vi "load_stepfile.vi"(8 "error in (no error)":errorcluster, 11 "_delayStageBase in":refnum<class "_delayStageBase.lvclass">) -> (0 "error out":errorcluster, 3 "_delayStageBase out":refnum<class "_delayStageBase.lvclass">)   [LabVIEW 2018, in "_delayStageBase.lvclass"]
uses:
  _delayStageBase.lvclass
  <vilib>/Utility/file.llb/Read Delimited Spreadsheet (DBL).vi
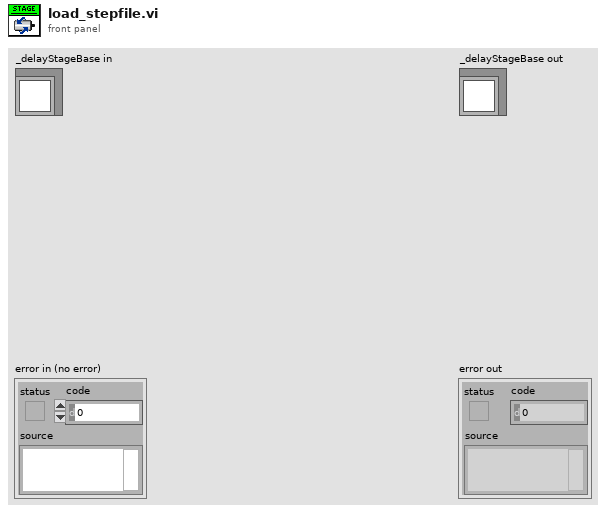
[diagram p1: front panel]
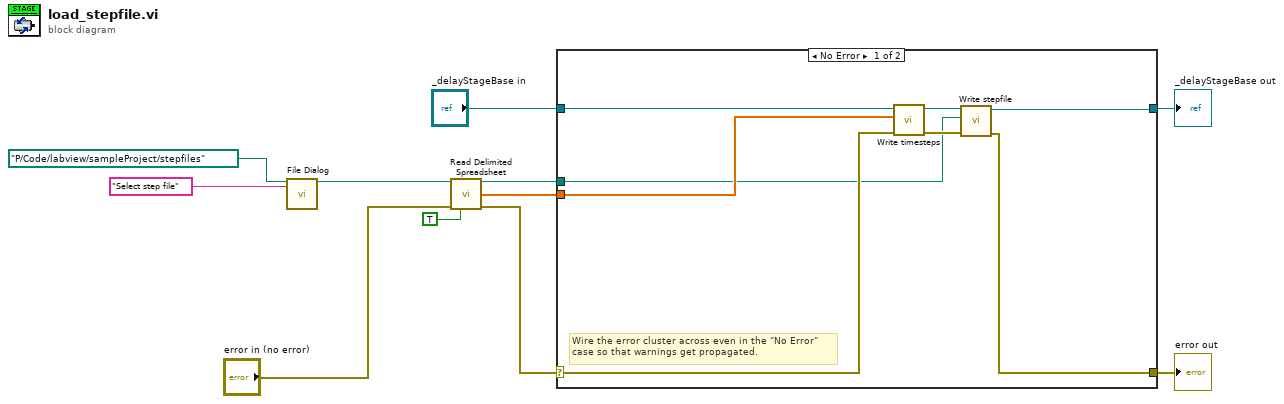
[diagram p0: block diagram]
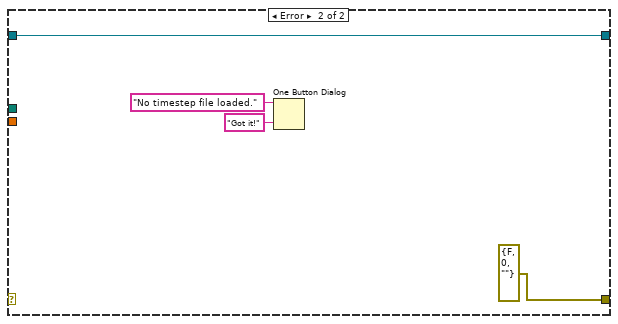
[diagram p2: hidden frame]
diagram:
  n1 = call "File Dialog"("start path"=path "P:/Code/labview/sampleProject/stepfiles", "prompt"="Select step file") -> ("selected path"=w3:path)  [unwired: 10 in, 3 out]
  n2 = call-poly <vilib>:"Read Delimited Spreadsheet.vi"("file path (dialog if empty)"=w3, "error in (no error)"="error in (no error)", "transpose? (F)"=TRUE) -> ("new file path (Not A Path if cancelled)"=w4:path, "first row"=w8:dbl[], "error out"=w5:errorcluster)  [unwired: 7 in, 3 out]
  n3 = case shown="No Error" w5 {
    selector: w5 -> [w18 _]
    tunnel: [w13 errorcluster {"status"=FALSE, "code"=0, "source"=""} ("error out")] -> w11
    tunnel: [w15 w23] -> w9
    tunnel: "_delayStageBase in" -> [w19 w23]
    tunnel: w8 -> [w17 _]
    tunnel: w4 -> [w12 _]
    frame No Error {
      # "Wire the error cluster across even in the \"No Error\"\ncase so that warnings get propagated."
      n4 = call-dynamic "Write timesteps.vi"("error in (no error)"=w18, "timesteps"=w17, "_delayStageBase in"=w19) -> ("error out"=w14:errorcluster, "_delayStageBase out"=w16:refnum<class "_delayStageBase.lvclass">)  [unwired: 7 in]
      n5 = call-dynamic "Write stepfile.vi"("error in (no error)"=w14, "stepfile"=w12, "_delayStageBase in"=w16) -> ("error out"=w13:errorcluster, "_delayStageBase out"=w15:refnum<class "_delayStageBase.lvclass">)  [unwired: 7 in]
    }
    frame Error {
      n6 = One Button Dialog(message="No timestep file loaded.", button name ("OK")="Got it!") -> ()  [unwired: 1 out]
    }
  }
  "error out" <- w11
  "_delayStageBase out" <- w9
